vi "sequence.vi"(0 "Elements@IC6":u16[](array[numeric])) -> (1 "Output Array":T2(array[cluster]), 2 "# of layers":i32, 3 "Start/Cancel":bool)   [LabVIEW 2012]
uses:
  elements.gbl
  <vilib>/Utility/VariantDataType/VariantType.lvlib
panel:
  out "Double click":i32
  in  "Clear all":bool
  out "Temp":T1 {"Temp Layer"."T (Å) / D (s)" min=0 format="%.1g"; "Temp Layer"."Elements" items=["none"]}
  in  "Clear layer":bool
  out "error out":errorcluster
  in  "error in (no error)":errorcluster
  in  "Scrollbar":i32(c297)
  in  "Layer Cluster":T3 {"T (Å) / D (s)" min=0 format="%.1g"; "Elements" items=["none"=0, "Se"=2, "Ti"=3, "Sn"=4]}
  in  "Cancel":bool
  in  "Start":bool
  in  "# of repeating units":i32=1 min=1
  in  "Repeats":i32=1 min=1 step=1
  in  "delete_cancel":bool
  in  "add_modify":bool
  in  "down":bool
  in  "up":bool
  in  "Sequence":i32(listbox)=-1
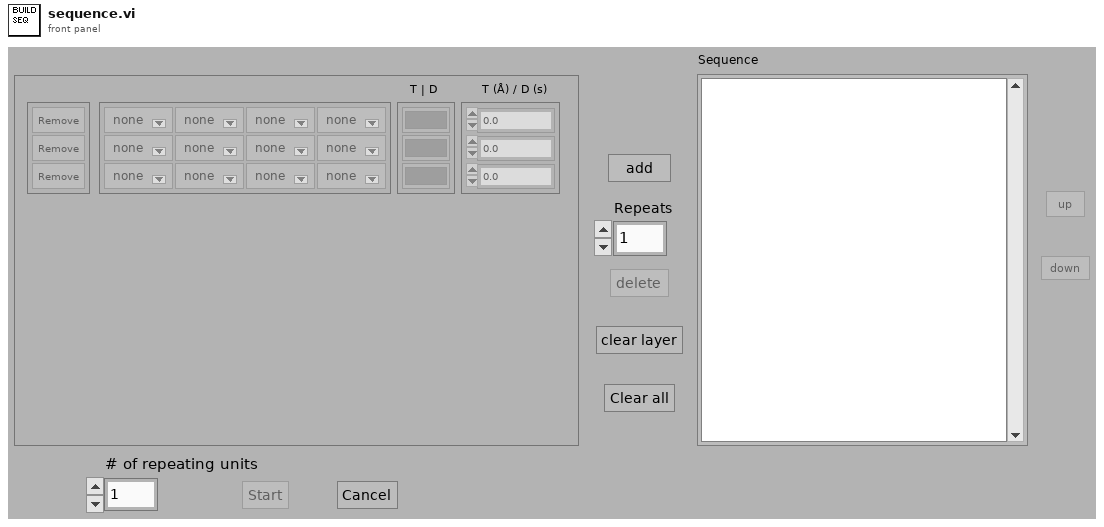
[diagram p1: front panel]
types:
  T1 = cluster{"Temp Layer":cluster{"Remove buttons":bool[], "Elements":u16[][], "T | D":bool[], "T (Å) / D (s)":sgl[]}, "Temp repeats":i32}
  T2 = cluster{"Elements":u16[][], "TD":bool[], "Value":sgl[], "Repeats":i32}[]
  T3 = cluster{"Remove buttons":bool[], "Elements":u16[][], "T | D":bool[], "T (Å) / D (s)":sgl[]}
  T4 = typedef "VariantType.lvlib/Type.ctl" = enum8{"Invalid Type", "Void", "I8", "I16", "I32", "I64", "U8", "U16", "U32", "U64", "Single Float", "Double Float", "Extended Float", "Single Complex", "Double Complex", "Extended Complex", "Enum U8", "Enum U16", "Enum U32", "Enum U64", "Single Float With Unit", "Double Float With Unit", "Extended Float With Unit", "Single Complex with Unit", "Double Complex with Unit", "Extended Complex with Unit", "Boolean", "String", "Path", "Picture", "Tag", "Array", "Cluster", "Variant", "LV Variant", "Waveform", "Timestamp", "Digital Waveform", "Digital Data", "ExpressData", "Refnum", "External Data", "VI", "Poly VI", "LabVIEW Class Instance", "Fixed Point"}
  T5 = cluster{"Layer Cluster":cluster{"Remove buttons":bool[], "Elements":u16[][], "T | D":bool[], "T (Å) / D (s)":sgl[]}, "Repeats":i32}
  T6 = cluster{"Elements":u16[][], "TD":bool[], "Value":sgl[], "Repeats":i32}
  T7 = cluster{bool[], "Elements":u16[][], "TD":bool[], "Value":sgl[]}
  T8 = typedef "LVStringsAndValuesArrayTypeDef_U16.ctl" = cluster{"String":string, "Value":u16}[]
  T9 = cluster{"Elements":u16[][], "T | D":bool[], "T (Å) / D (s)":sgl[]}
  T10 = cluster{"Elements":u16[][], "T|D":bool[], "T (Å) / D (s)":sgl[], "Repeats":i32}
  T11 = cluster{"Elements":u16[][], "T|D":bool[], "T (Å) / D (s)":sgl[], "Repeats":i32}[]
  T12 = cluster{cluster{bool[], u16[][], bool[], sgl[]}, i32}
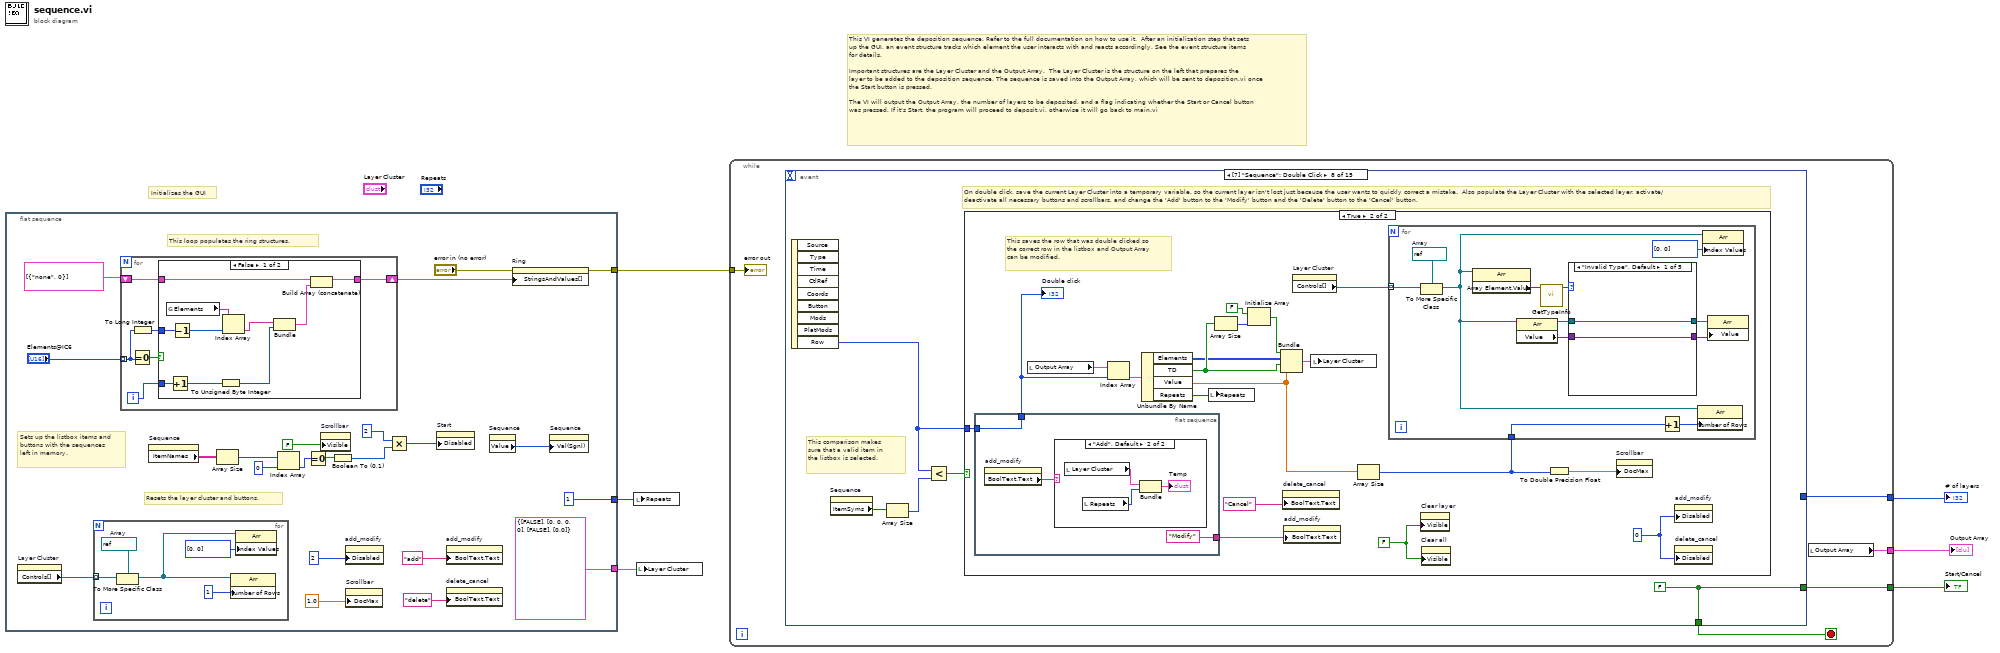
[diagram p0: block diagram]
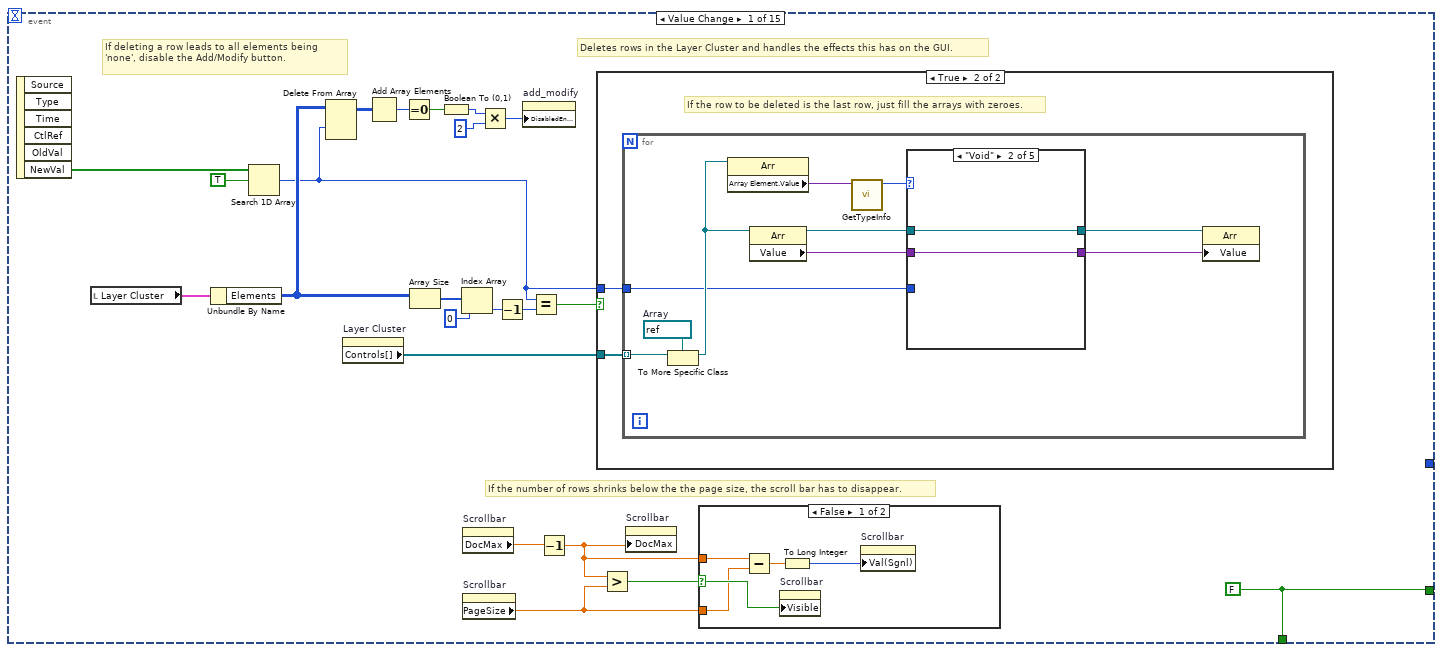
[diagram p2: hidden frame]
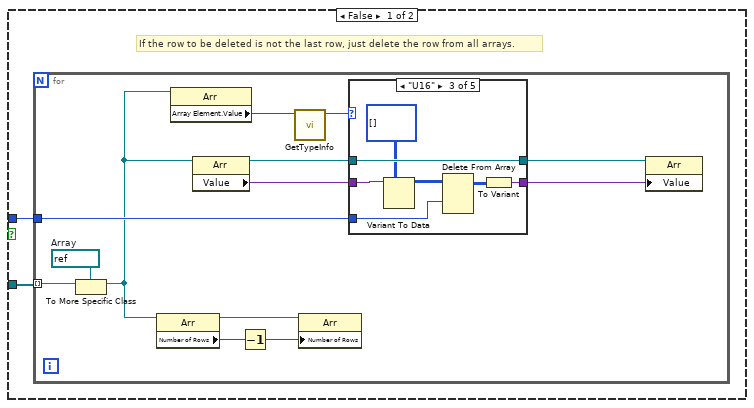
[diagram p4: hidden frame]
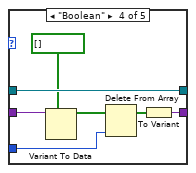
[diagram p7: hidden frame]
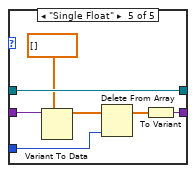
[diagram p8: hidden frame]
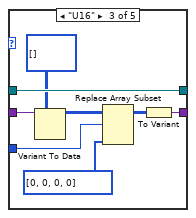
[diagram p10: hidden frame]
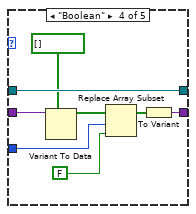
[diagram p11: hidden frame]
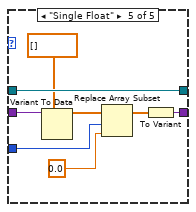
[diagram p12: hidden frame]
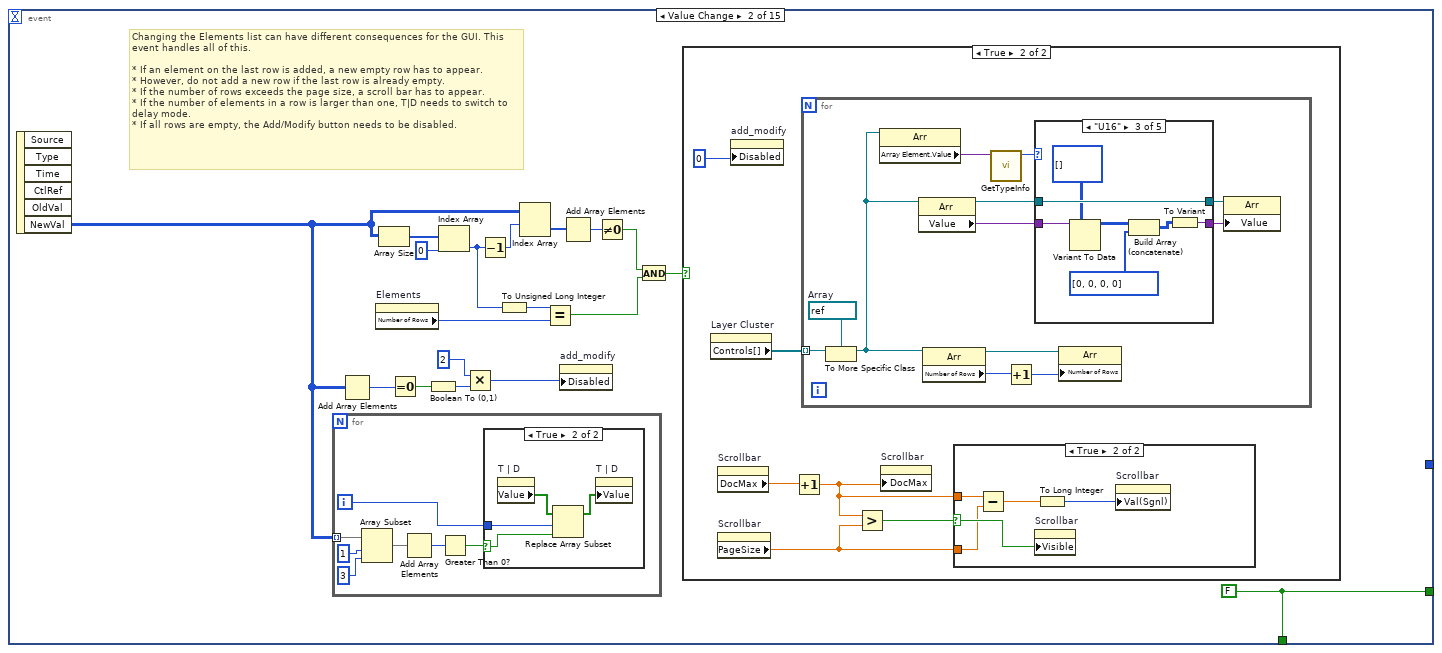
[diagram p13: hidden frame]
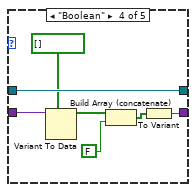
[diagram p19: hidden frame]
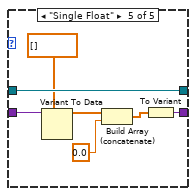
[diagram p20: hidden frame]
diagram:
  # "Initializes the GUI"
  # "This VI generates the deposition sequence. Refer to the full documentation on how to use it.  After an initialization step that sets up the GUI, an event structure tracks which element the user interacts with and reacts accordingly. See the event structure items for details.\n\nImportant structures are the Layer Cluster and the Output Array.  The Layer Cluster is the structure on the left that prepares the layer to be added to the deposition sequence. The sequence is saved into the Output Array, which will be sent to deposition.vi once the Start button is pressed.\n\nThe VI will output the Output Array, the number of layers to be deposited, and a flag indicating whether the Start or Cancel button was pressed. If it's Start, the program will proceed to deposit.vi, otherwise it will go back to main.vi"
  n1 = flat-sequence {
    tunnel: [w28] -> w6
    tunnel: [cluster{bool[], u16[][], bool[], sgl[]} {[FALSE], [[0, 0, 0, 0]], [FALSE], [0.0]}] -> w3
    tunnel: [1] -> w2
    frame #0 {
      # "Sets up the listbox items and buttons with the sequences left in memory."
      # "Resets the layer cluster and buttons."
      # "This loop populates the ring structures."
      n2 = property on="Layer Cluster" class="Clust (strict)"() -> ("Controls[]"=w24:refnum<vi>[])  [unwired: 2 in, 2 out]
      n3 = for {
        tunnel: w24 -> [w32] mode=indexing
        w33 = refnum<vi> refnum  # Array
        n4 = To More Specific Class(target class=w33, reference=w32) -> (specific class reference=w30:refnum<vi>)  [unwired: 1 in, 1 out]
        n5 = property class="Arr"(reference=w30, "Number of Rows"=u32 1) -> ()  [unwired: 1 in, 2 out]
        n6 = property class="Arr"(reference=w30, "Index Values"=u32[] [0, 0]) -> ()  [unwired: 1 in, 2 out]
      }
      n7 = for {
        shift-right: [w38] -> w25
        shift-left: cluster{string, i32}[] [{"none", 0}] -> [w39]
        tunnel: "Elements@IC6" -> [w35] mode=indexing
        i -> [w36]
        n8 = Equal To 0?(x=w35) -> (x = 0?=w37:bool)
        n9 = To Long Integer(number=w35) -> (32bit integer=w34:i32)
        n10 = case shown="False" w37 {
          tunnel: w39 -> [w49 w50]
          tunnel: [w48 w50] -> w38
          tunnel: w36 -> [w47 _]
          tunnel: w34 -> [w45 _]
          frame False {
            n11 = global read "elements.gbl" "Elements"() -> (w46:string[])
            n12 = Increment(x=w47) -> (x+1=w43:i32)
            n13 = Decrement(x=w45) -> (x-1=w40:i32)
            n14 = To Unsigned Byte Integer(number=w43) -> (unsigned 8bit integer=w42:u8)
            n15 = Index Array(array=w46, index=w40) -> (element=w44:string)
            n16 = Bundle("String"=w44, w42) -> (w41:cluster{"String":string, u8})  [unwired: 1 in]
            n17 = Build Array (concatenate)(w49, w41) -> (w48:cluster{"String":string, i32}[])
          }
          frame True {
          }
        }
      }
      n18 = property on="Sequence" class="MCListbox (strict)"() -> ("ItemNames"=w22:string[][])  [unwired: 2 in, 2 out]
      n19 = Array Size(array=w22) -> (size(s)=w21:i32[])
      n20 = Index Array(array=w21, index=0) -> (element=w19:i32)
      n21 = Equal To 0?(x=w19) -> (x = 0?=w18:bool)
      n22 = property on="Scrollbar" class="Scroll (strict)"("Visible"=FALSE) -> ()  [unwired: 2 in, 2 out]
      n23 = Boolean To (0,1)(Boolean=w18) -> (0, 1=w7:i16)
      n24 = property on="add_modify" class="Bool"("Disabled"=2) -> ()  [unwired: 2 in, 2 out]
      n25 = property on="Scrollbar" class="Scroll (strict)"("DocMax"=1.0) -> ()  [unwired: 2 in, 2 out]
      n26 = Multiply(x=i16 2, y=w7) -> (x*y=w16:i16)
      n27 = property on="Start" class="Bool"("Disabled"=w16) -> ()  [unwired: 2 in, 2 out]
      n28 = property on="add_modify" class="Bool"("BoolText.Text"="add") -> ()  [unwired: 2 in, 2 out]
      n29 = property on="delete_cancel" class="Bool"("BoolText.Text"="delete") -> ()  [unwired: 2 in, 2 out]
      n30 = property on="Sequence" class="MCListbox (strict)"() -> ("Value"=w11:i32)  [unwired: 2 in, 2 out]
      n31 = property on="Ring" class="Ring (strict)"(error in="error in (no error)", "StringsAndValues[]"=w25) -> (error out=w28:errorcluster)  [unwired: 1 in, 1 out]
      n32 = property on="Sequence" class="MCListbox (strict)"("Val(Sgnl)"=w11) -> ()  [unwired: 2 in, 2 out]
    }
  }
  n33 = local write "Repeats"(w2) -> ()
  n34 = local write "Layer Cluster"(w3) -> ()
  n35 = while {
    tunnel: w6 -> [w55]
    tunnel: [w54] -> w5
    tunnel: [w51] -> w4
    tunnel: [w52] -> w1
    stop <- w53 stop-if-true
    n36 = event shown="[7] \"Sequence\": Double Click" {
      selector: _ -> [_ _ _ _ _ _ _ _ _ _ _ _ _ _ _]
      dyn-events: _ -> [_ _ _ _ _ _ _ _ _ _ _ _ _ _ _]
      timeout: _ -> [_ _ _ _ _ _ _ _ _ _ _ _ _ _ _]
      tunnel: [w65 w170 w248 w259 w268 "Cancel" w274 w295 w368 w379 w399 w466 w495 w512 w518] -> w53
      tunnel: [w65 w170 w248 w259 w268 w271 w274 w295 w368 w379 w399 w466 w495 w512 w518] -> w54
      tunnel: [_ _ _ _ "# of repeating units" _ _ _ _ _ _ _ _ _ _] -> w51
      event "Layer Cluster.Remove buttons": Value Change {
        w65 = FALSE
        # "If deleting a row leads to all elements being 'none', disable the Add/Modify button."
        # "If the number of rows shrinks below the the page size, the scroll bar has to disappear."
        # "Deletes rows in the Layer Cluster and handles the effects this has on the GUI."
        n37 = event-data() -> ("NewVal"=w76:bool[])  [unwired: 1 in, 5 out]
        n38 = local read "Layer Cluster"() -> (w64:T3)
        n39 = Unbundle By Name(w64) -> ("Elements"=w57:u16[][])
        n40 = Search 1D Array(1D array=w76, element=TRUE) -> (index of element=w56:i32)  [unwired: 1 in]
        n41 = Delete From Array(array=w57, index (row)=w56) -> (array with subset deleted=w58:u16[][])  [unwired: 2 in, 1 out]
        n42 = property on="Layer Cluster" class="Clust (strict)"() -> ("Controls[]"=w75:refnum<vi>[])  [unwired: 2 in, 2 out]
        n43 = Add Array Elements(numeric array=w58) -> (sum=w63:u16)
        n44 = Equal To 0?(x=w63) -> (x = 0?=w62:bool)
        n45 = Array Size(array=w57) -> (size(s)=w74:i32[])
        n46 = Boolean To (0,1)(Boolean=w62) -> (0, 1=w60:i16)
        n47 = Index Array(array=w74, index=0) -> (element=w72:i32)
        n48 = property on="Scrollbar" class="Scroll (strict)"() -> ("DocMax"=w69:dbl)  [unwired: 2 in, 2 out]
        n49 = property on="Scrollbar" class="Scroll (strict)"() -> ("PageSize"=w66:dbl)  [unwired: 2 in, 2 out]
        n50 = Multiply(x=w60, y=2) -> (x*y=w59:i32)
        n51 = Decrement(x=w72) -> (x-1=w70:i32)
        n52 = property on="add_modify" class="Bool"("DisabledEnum"=w59) -> ()  [unwired: 2 in, 2 out]
        n53 = Equal?(x=w56, y=w70) -> (x = y?=w71:bool)
        n54 = Decrement(x=w69) -> (x-1=w68:dbl)
        n55 = case shown="True" w71 {
          tunnel: w75 -> [w84 w124]
          tunnel: w56 -> [w83 w123]
          frame False {
            # "If the row to be deleted is not the last row, just delete the row from all arrays."
            n56 = for {
              tunnel: w84 -> [w93] mode=indexing
              tunnel: w83 -> [w91]
              w97 = refnum<vi> refnum  # Array
              n57 = To More Specific Class(target class=w97, reference=w93) -> (specific class reference=w89:refnum<vi>)  [unwired: 1 in, 1 out]
              n58 = property class="Arr"(reference=w89) -> (reference out=w94:refnum<vi>, "Number of Rows"=w96:u32)  [unwired: 1 in, 1 out]
              n59 = property class="Arr"(reference=w89) -> ("Array Element.Value"=w90:variant)  [unwired: 1 in, 2 out]
              n60 = property class="Arr"(reference=w89) -> (reference out=w86:refnum<vi>, "Value"=w88:variant)  [unwired: 1 in, 1 out]
              n61 = Decrement(x=w96) -> (x-1=w95:u32)
              n62 = call <vilib>:"GetTypeInfo.vi"("Variant"=w90) -> ("Type Enum"=w92:T4)  [unwired: 6 in, 4 out]
              n63 = property class="Arr"(reference=w94, "Number of Rows"=w95) -> ()  [unwired: 1 in, 2 out]
              n64 = case shown="\"U16\"" w92 {
                tunnel: w91 -> [_ _ w102 w114 w121]
                tunnel: w88 -> [w99 w101 w106 w112 w119]
                tunnel: [w99 w101 w107 w109 w118] -> w87
                tunnel: w86 -> [w98 w100 w108 w115 w122]
                tunnel: [w98 w100 w108 w115 w122] -> w85
                frame "Invalid Type", Default {
                }
                frame "Void" {
                }
                frame "U16" {
                  n65 = Variant To Data(type=u16[][] [], Variant=w106) -> (data=w104:u16[][])  [unwired: 1 in, 1 out]
                  n66 = Delete From Array(array=w104, index (row)=w102) -> (array with subset deleted=w105:u16[][])  [unwired: 2 in, 1 out]
                  n67 = To Variant(anything=w105) -> (Variant=w107:variant)
                }
                frame "Boolean" {
                  n68 = Variant To Data(type=bool[] [], Variant=w112) -> (data=w113:bool[])  [unwired: 1 in, 1 out]
                  n69 = Delete From Array(array=w113, index=w114) -> (array with subset deleted=w110:bool[])  [unwired: 1 in, 1 out]
                  n70 = To Variant(anything=w110) -> (Variant=w109:variant)
                }
                frame "Single Float" {
                  n71 = Variant To Data(type=sgl[] [], Variant=w119) -> (data=w120:sgl[])  [unwired: 1 in, 1 out]
                  n72 = Delete From Array(array=w120, index=w121) -> (array with subset deleted=w117:sgl[])  [unwired: 1 in, 1 out]
                  n73 = To Variant(anything=w117) -> (Variant=w118:variant)
                }
              }
              n74 = property class="Arr"(reference=w85, "Value"=w87) -> ()  [unwired: 1 in, 2 out]
            }
          }
          frame True {
            # "If the row to be deleted is the last row, just fill the arrays with zeroes."
            n75 = for {
              tunnel: w124 -> [w127] mode=indexing
              tunnel: w123 -> [w125]
              w128 = refnum<vi> refnum  # Array
              n76 = To More Specific Class(target class=w128, reference=w127) -> (specific class reference=w126:refnum<vi>)  [unwired: 1 in, 1 out]
              n77 = property class="Arr"(reference=w126) -> ("Array Element.Value"=w133:variant)  [unwired: 1 in, 2 out]
              n78 = property class="Arr"(reference=w126) -> (reference out=w129:refnum<vi>, "Value"=w132:variant)  [unwired: 1 in, 1 out]
              n79 = call <vilib>:"GetTypeInfo.vi"("Variant"=w133) -> ("Type Enum"=w134:T4)  [unwired: 6 in, 4 out]
              n80 = case shown="\"Void\"" w134 {
                tunnel: w125 -> [_ _ w140 w153 w161]
                tunnel: w132 -> [w136 w138 w144 w151 w159]
                tunnel: [w136 w138 w145 w148 w158] -> w131
                tunnel: w129 -> [w135 w137 w146 w154 w162]
                tunnel: [w135 w137 w146 w154 w162] -> w130
                frame "Invalid Type", Default {
                }
                frame "Void" {
                }
                frame "U16" {
                  n81 = Variant To Data(type=u16[][] [], Variant=w144) -> (data=w142:u16[][])  [unwired: 1 in, 1 out]
                  n82 = Replace Array Subset(array=w142, new element=u16[] [0, 0, 0, 0], index (row)=w140) -> (w143:u16[][])  [unwired: 1 in]
                  n83 = To Variant(anything=w143) -> (Variant=w145:variant)
                }
                frame "Boolean" {
                  n84 = Variant To Data(type=bool[] [], Variant=w151) -> (data=w152:bool[])  [unwired: 1 in, 1 out]
                  n85 = Replace Array Subset(array=w152, new element=FALSE, index=w153) -> (w149:bool[])
                  n86 = To Variant(anything=w149) -> (Variant=w148:variant)
                }
                frame "Single Float" {
                  n87 = Variant To Data(type=sgl[] [], Variant=w159) -> (data=w160:sgl[])  [unwired: 1 in, 1 out]
                  n88 = Replace Array Subset(array=w160, new element=sgl 0.0, index=w161) -> (w157:sgl[])
                  n89 = To Variant(anything=w157) -> (Variant=w158:variant)
                }
              }
              n90 = property class="Arr"(reference=w130, "Value"=w131) -> ()  [unwired: 1 in, 2 out]
            }
          }
        }
        n91 = Greater?(x=w68, y=w66) -> (0:w67:bool)
        n92 = property on="Scrollbar" class="Scroll (strict)"("DocMax"=w68) -> ()  [unwired: 2 in, 2 out]
        n93 = case shown="False" w67 {
          selector: w67 -> [w82 _]
          tunnel: w68 -> [w80 _]
          tunnel: w66 -> [w79 _]
          frame False {
            n94 = Subtract(x=w80, y=w79) -> (x-y=w78:dbl)
            n95 = property on="Scrollbar" class="Scroll (strict)"("Visible"=w82) -> ()  [unwired: 2 in, 2 out]
            n96 = To Long Integer(number=w78) -> (32bit integer=w81:i32)
            n97 = property on="Scrollbar" class="Scroll (strict)"("Val(Sgnl)"=w81) -> ()  [unwired: 2 in, 2 out]
          }
          frame True {
          }
        }
      }
      event "Layer Cluster.Elements": Value Change {
        w170 = FALSE
        # "Changing the Elements list can have different consequences for the GUI. This event handles all of this.\n\n* If an element on the last row is added, a new empty row has to appear.\n* However, do not add a new row if the last row is already empty.\n* If the number of rows exceeds the page size, a scroll bar has to appear.\n* If the number of elements in a row is larger than one, T|D needs to switch to delay mode.\n* If all rows are empty, the Add/Modify button needs to be disabled."
        n98 = event-data() -> ("NewVal"=w164:u16[][])  [unwired: 1 in, 5 out]
        n99 = for {
          tunnel: w164 -> [w187] mode=indexing
          i -> [w182]
          n100 = Array Subset(array=w187, index=1, length=3) -> (w184:u16[])
          n101 = Add Array Elements(numeric array=w184) -> (sum=w183:u16)
          n102 = Greater Than 0?(x=w183) -> (x > 0?=w181:bool)
          n103 = case shown="True" w181 {
            selector: w181 -> [_ w188]
            tunnel: w182 -> [_ w189]
            frame False {
            }
            frame True {
              n104 = property on="T | D" class="Arr (strict)"() -> ("Value"=w191:bool[])  [unwired: 2 in, 2 out]
              n105 = Replace Array Subset(array=w191, new element=w188, index=w189) -> (w190:bool[])
              n106 = property on="T | D" class="Arr (strict)"("Value"=w190) -> ()  [unwired: 2 in, 2 out]
            }
          }
        }
        n107 = Add Array Elements(numeric array=w164) -> (sum=w169:u16)
        n108 = property on="Elements" class="Arr (strict)"() -> ("Number of Rows"=w171:u32)  [unwired: 2 in, 2 out]
        n109 = Array Size(array=w164) -> (size(s)=w180:i32[])
        n110 = Equal To 0?(x=w169) -> (x = 0?=w168:bool)
        n111 = Boolean To (0,1)(Boolean=w168) -> (0, 1=w167:i16)
        n112 = Index Array(array=w180, index=0) -> (element=w172:i32)
        n113 = Multiply(x=i16 2, y=w167) -> (x*y=w165:i16)
        n114 = Decrement(x=w172) -> (x-1=w176:i32)
        n115 = To Unsigned Long Integer(number=w172) -> (unsigned 32bit integer=w163:u32)
        n116 = Index Array(array=w164, index (row)=w176) -> (element=w178:u16[])  [unwired: 1 in]
        n117 = Equal?(x=w163, y=w171) -> (x = y?=w173:bool)
        n118 = property on="add_modify" class="Bool"("Disabled"=w165) -> ()  [unwired: 2 in, 2 out]
        n119 = Add Array Elements(numeric array=w178) -> (sum=w177:u16)
        n120 = Not Equal To 0?(x=w177) -> (x != 0?=w174:bool)
        n121 = And(x=w174, y=w173) -> (x .and. y?=w175:bool)
        n122 = case shown="True" w175 {
          frame False {
            # "Last row is empty, so do not add another empty row."
          }
          frame True {
            n123 = property on="Layer Cluster" class="Clust (strict)"() -> ("Controls[]"=w197:refnum<vi>[])  [unwired: 2 in, 2 out]
            n124 = property on="Scrollbar" class="Scroll (strict)"() -> ("DocMax"=w196:dbl)  [unwired: 2 in, 2 out]
            n125 = property on="Scrollbar" class="Scroll (strict)"() -> ("PageSize"=w193:dbl)  [unwired: 2 in, 2 out]
            n126 = property on="add_modify" class="Bool"("Disabled"=u16 0) -> ()  [unwired: 2 in, 2 out]
            n127 = Increment(x=w196) -> (x+1=w195:dbl)
            n128 = for {
              tunnel: w197 -> [w214] mode=indexing
              w213 = refnum<vi> refnum  # Array
              n129 = To More Specific Class(target class=w213, reference=w214) -> (specific class reference=w204:refnum<vi>)  [unwired: 1 in, 1 out]
              n130 = property class="Arr"(reference=w204) -> ("Array Element.Value"=w203:variant)  [unwired: 1 in, 2 out]
              n131 = property class="Arr"(reference=w204) -> (reference out=w207:refnum<vi>, "Value"=w206:variant)  [unwired: 1 in, 1 out]
              n132 = property class="Arr"(reference=w204) -> (reference out=w212:refnum<vi>, "Number of Rows"=w210:u32)  [unwired: 1 in, 1 out]
              n133 = call <vilib>:"GetTypeInfo.vi"("Variant"=w203) -> ("Type Enum"=w205:T4)  [unwired: 6 in, 4 out]
              n134 = Increment(x=w210) -> (x+1=w211:u32)
              n135 = case shown="\"U16\"" w205 {
                tunnel: w206 -> [w216 w218 w223 w230 w237]
                tunnel: [w216 w218 w224 w227 w236] -> w208
                tunnel: w207 -> [w215 w217 w225 w232 w239]
                tunnel: [w215 w217 w225 w232 w239] -> w209
                frame "Invalid Type", Default {
                }
                frame "Void" {
                }
                frame "U16" {
                  n136 = Variant To Data(type=u16[][] [], Variant=w223) -> (data=w219:u16[][])  [unwired: 1 in, 1 out]
                  n137 = Build Array (concatenate)(w219, u16[] [0, 0, 0, 0]) -> (w222:u16[][])
                  n138 = To Variant(anything=w222) -> (Variant=w224:variant)
                }
                frame "Boolean" {
                  n139 = Variant To Data(type=bool[] [], Variant=w230) -> (data=w231:bool[])  [unwired: 1 in, 1 out]
                  n140 = Build Array (concatenate)(w231, FALSE) -> (w228:bool[])
                  n141 = To Variant(anything=w228) -> (Variant=w227:variant)
                }
                frame "Single Float" {
                  n142 = Variant To Data(type=sgl[] [], Variant=w237) -> (data=w238:sgl[])  [unwired: 1 in, 1 out]
                  n143 = Build Array (concatenate)(w238, sgl 0.0) -> (w235:sgl[])
                  n144 = To Variant(anything=w235) -> (Variant=w236:variant)
                }
              }
              n145 = property class="Arr"(reference=w212, "Number of Rows"=w211) -> ()  [unwired: 1 in, 2 out]
              n146 = property class="Arr"(reference=w209, "Value"=w208) -> ()  [unwired: 1 in, 2 out]
            }
            n147 = Greater?(x=w195, y=w193) -> (0:w194:bool)
            n148 = property on="Scrollbar" class="Scroll (strict)"("DocMax"=w195) -> ()  [unwired: 2 in, 2 out]
            n149 = case shown="True" w194 {
              selector: w194 -> [_ w202]
              tunnel: w195 -> [_ w201]
              tunnel: w193 -> [_ w198]
              frame False {
              }
              frame True {
                n150 = Subtract(x=w201, y=w198) -> (x-y=w199:dbl)
                n151 = property on="Scrollbar" class="Scroll (strict)"("Visible"=w202) -> ()  [unwired: 2 in, 2 out]
                n152 = To Long Integer(number=w199) -> (32bit integer=w200:i32)
                n153 = property on="Scrollbar" class="Scroll (strict)"("Val(Sgnl)"=w200) -> ()  [unwired: 2 in, 2 out]
              }
            }
          }
        }
      }
      event "Layer Cluster.T | D": Value Change {
        w248 = FALSE
        # "Prevents going to thickness mode when more than one element is in the layer."
        n154 = event-data() -> ("OldVal"=w253:bool[], "NewVal"=w252:bool[])  [unwired: 1 in, 4 out]
        n155 = Not Equal?(x=w253, y=w252) -> (x != y?=w251:bool[])
        n156 = Search 1D Array(1D array=w251, element=TRUE) -> (index of element=w246:i32)  [unwired: 1 in]
        n157 = local read "Layer Cluster"() -> (w249:T3)
        n158 = Unbundle By Name(w249) -> ("Elements"=w247:u16[][])
        n159 = Index Array(array=w247, index (row)=w246) -> (element=w245:u16[])  [unwired: 1 in]
        n160 = Not Equal To 0?(x=w245) -> (x != 0?=w244:bool[])
        n161 = Boolean To (0,1)(Boolean=w244) -> (0, 1=w243:i16[])
        n162 = Add Array Elements(numeric array=w243) -> (sum=w241:i16)
        n163 = Less?(x=i16 1, y=w241) -> (x < y?=w242:bool)
        n164 = case shown="True" w242 {
          selector: w242 -> [_ w254]
          tunnel: w246 -> [_ w255]
          frame False {
          }
          frame True {
            n165 = property on="T | D" class="Arr (strict)"() -> ("Value"=w257:bool[])  [unwired: 2 in, 2 out]
            n166 = Replace Array Subset(array=w257, new element=w254, index=w255) -> (w256:bool[])
            n167 = property on="T | D" class="Arr (strict)"("Value"=w256) -> ()  [unwired: 2 in, 2 out]
          }
        }
      }
      event "Scrollbar": Value Change {
        w259 = FALSE
        # "Moves the layer cluster with the scrollbar."
        n168 = event-data() -> ("NewVal"=w258:i32)  [unwired: 1 in, 5 out]
        n169 = property on="Layer Cluster" class="Clust (strict)"() -> ("Controls[]"=w262:refnum<vi>[])  [unwired: 2 in, 2 out]
        n170 = Build Array(w258, 0) -> (w260:i32[])
        n171 = for {
          tunnel: w262 -> [w266] mode=indexing
          tunnel: w260 -> [w264]
          w267 = refnum<vi> refnum  # Array
          n172 = To Unsigned Long Integer(number=w264) -> (unsigned 32bit integer=w263:u32[])
          n173 = To More Specific Class(target class=w267, reference=w266) -> (specific class reference=w265:refnum<vi>)  [unwired: 1 in, 1 out]
          n174 = property class="Arr"(reference=w265, "Index Values"=w263) -> ()  [unwired: 1 in, 2 out]
        }
      }
      event "Start": Value Change {
        w268 = TRUE
        # "Quits the VI and sends a True (Start) signal and the number of layers to main.vi"
        n175 = event-data() -> ()  [unwired: 1 in, 6 out]
      }
      event "Cancel": Value Change {
        # "Quits the VI and sends a False (Cancel) signal to main.vi"
        n176 = event-data() -> ()  [unwired: 1 in, 6 out]
        n177 = Not(x="Cancel") -> (.not. x?=w271:bool)
      }
      event "Sequence": Value Change {
        w274 = FALSE
        # "Activates/dectivates buttons, depending on which item in the listbox is selected.\n\n0: First item selected, disable the 'up' button.\n< 0: No item selected, disable the 'delete' button.\n= length of items - 1: Last item selected, disable 'down' button."
        n178 = event-data() -> ("NewVal"=w275:i32)  [unwired: 1 in, 5 out]
        n179 = property on="Sequence" class="MCListbox (strict)"() -> ("ItemSyms"=w280:i32[])  [unwired: 2 in, 2 out]
        n180 = Array Size(array=w280) -> (size(s)=w272:i32)
        n181 = Decrement(x=w272) -> (x-1=w273:i32)
        n182 = Equal To 0?(x=w275) -> (x = 0?=w283:bool)
        n183 = Less Than 0?(x=w275) -> (x < 0?=w277:bool)
        n184 = Equal?(x=w275, y=w273) -> (x = y?=w281:bool)
        n185 = Or(x=w283, y=w277) -> (x .or. y?=w284:bool)
        n186 = Or(x=w277, y=w281) -> (x .or. y?=w282:bool)
        n187 = Boolean To (0,1)(Boolean=w277) -> (0, 1=w278:i16)
        n188 = Boolean To (0,1)(Boolean=w284) -> (0, 1=w290:i16)
        n189 = Boolean To (0,1)(Boolean=w282) -> (0, 1=w287:i16)
        n190 = Multiply(x=i16 2, y=w290) -> (x*y=w288:i16)
        n191 = Multiply(x=i16 2, y=w278) -> (x*y=w276:i16)
        n192 = Multiply(x=i16 2, y=w287) -> (x*y=w285:i16)
        n193 = property on="up" class="Bool"("Disabled"=w288) -> ()  [unwired: 2 in, 2 out]
        n194 = property on="delete_cancel" class="Bool"("Disabled"=w276) -> ()  [unwired: 2 in, 2 out]
        n195 = property on="down" class="Bool"("Disabled"=w285) -> ()  [unwired: 2 in, 2 out]
      }
      event "Sequence": Double Click {
        w295 = FALSE
        # "On double click, save the current Layer Cluster into a temporary variable, so the current layer isn't lost just because the user wants to quickly correct a mistake.  Also populate the Layer Cluster with the selected layer, activate/deactivate all necessary buttons and scrollbars, and change the 'Add' button to the 'Modify' button and the 'Delete' button to the 'Cancel' button."
        # "This comparison makes sure that a valid item in the listbox is selected."
        n196 = event-data() -> ("Row"=w291:i32)  [unwired: 1 in, 8 out]
        n197 = property on="Sequence" class="MCListbox (strict)"() -> ("ItemSyms"=w294:i32[])  [unwired: 2 in, 2 out]
        n198 = Array Size(array=w294) -> (size(s)=w292:i32)
        n199 = Less?(x=w291, y=w292) -> (x < y?=w293:bool)
        n200 = case shown="True" w293 {
          tunnel: w291 -> [_ w302]
          frame False {
          }
          frame True {
            w305 = FALSE
            w298 = 0
            # "This saves the row that was double clicked so the correct row in the listbox and Output Array can be modified."
            n201 = flat-sequence {
              tunnel: w302 -> [w353]
              tunnel: [w353] -> w297
              tunnel: ["Modify"] -> w296
              frame #0 {
                n202 = property on="add_modify" class="Bool"() -> ("BoolText.Text"=w354:string)  [unwired: 2 in, 2 out]
                n203 = case shown="\"Add\", Default" w354 {
                  frame "Modify" {
                  }
                  frame "Add", Default {
                    n204 = local read "Layer Cluster"() -> (w356:T3)
                    n205 = local read "Repeats"() -> (w355:i32)
                    n206 = Bundle("Layer Cluster"=w356, "Repeats"=w355) -> (→"Temp":T5)  [unwired: 1 in]
                  }
                }
              }
            }
            n207 = local read "Output Array"() -> (w313:T2)
            n208 = Index Array(array=w313, index=w297) -> (element=w312:T6)
            n209 = Unbundle By Name(w312) -> ("Elements"=w301:u16[][], "TD"=w306:bool[], "Value"=w304:sgl[], "Repeats"=w311:i32)
            n210 = local write "Repeats"(w311) -> ()
            n211 = Array Size(array=w306) -> (size(s)=w309:i32)
            n212 = Initialize Array(FALSE, w309) -> (w308:bool[])
            n213 = Bundle(w308, "Elements"=w301, "TD"=w306, "Value"=w304) -> (w307:T7)  [unwired: 1 in]
            n214 = property on="delete_cancel" class="Bool"("BoolText.Text"="Cancel") -> ()  [unwired: 2 in, 2 out]
            n215 = property on="add_modify" class="Bool"("BoolText.Text"=w296) -> ()  [unwired: 2 in, 2 out]
            n216 = property on="Layer Cluster" class="Clust (strict)"() -> ("Controls[]"=w300:refnum<vi>[])  [unwired: 2 in, 2 out]
            n217 = local write "Layer Cluster"(w307) -> ()
            n218 = Array Size(array=w304) -> (size(s)=w299:i32)
            n219 = for {
              tunnel: w300 -> [w325] mode=indexing
              tunnel: w299 -> [w323]
              w326 = refnum<vi> refnum  # Array
              n220 = To More Specific Class(target class=w326, reference=w325) -> (specific class reference=w315:refnum<vi>)  [unwired: 1 in, 1 out]
              n221 = property class="Arr"(reference=w315) -> ("Array Element.Value"=w317:variant)  [unwired: 1 in, 2 out]
              n222 = property class="Arr"(reference=w315) -> (reference out=w318:refnum<vi>, "Value"=w319:variant)  [unwired: 1 in, 1 out]
              n223 = call <vilib>:"GetTypeInfo.vi"("Variant"=w317) -> ("Type Enum"=w316:T4)  [unwired: 6 in, 4 out]
              n224 = case shown="\"Invalid Type\", Default" w316 {
                tunnel: w319 -> [w328 w330 w335 w342 w349]
                tunnel: [w328 w330 w336 w339 w348] -> w320
                tunnel: w318 -> [w327 w329 w337 w344 w351]
                tunnel: [w327 w329 w337 w344 w351] -> w321
                frame "Invalid Type", Default {
                }
                frame "Void" {
                }
                frame "U16" {
                  n225 = Variant To Data(type=u16[][] [], Variant=w335) -> (data=w333:u16[][])  [unwired: 1 in, 1 out]
                  n226 = Build Array (concatenate)(w333, u16[] [0, 0, 0, 0]) -> (w334:u16[][])
                  n227 = To Variant(anything=w334) -> (Variant=w336:variant)
                }
                frame "Boolean" {
                  n228 = Variant To Data(type=bool[] [], Variant=w342) -> (data=w343:bool[])  [unwired: 1 in, 1 out]
                  n229 = Build Array (concatenate)(w343, FALSE) -> (w340:bool[])
                  n230 = To Variant(anything=w340) -> (Variant=w339:variant)
                }
                frame "Single Float" {
                  n231 = Variant To Data(type=sgl[] [], Variant=w349) -> (data=w350:sgl[])  [unwired: 1 in, 1 out]
                  n232 = Build Array (concatenate)(w350, sgl 0.0) -> (w347:sgl[])
                  n233 = To Variant(anything=w347) -> (Variant=w348:variant)
                }
              }
              n234 = Increment(x=w323) -> (x+1=w322:i32)
              n235 = property class="Arr"(reference=w315, "Number of Rows"=w322) -> ()  [unwired: 1 in, 2 out]
              n236 = property class="Arr"(reference=w315, "Index Values"=i32[] [0, 0]) -> ()  [unwired: 1 in, 2 out]
              n237 = property class="Arr"(reference=w321, "Value"=w320) -> ()  [unwired: 1 in, 2 out]
            }
            n238 = property on="Clear layer" class="Bool"("Visible"=w305) -> ()  [unwired: 2 in, 2 out]
            n239 = property on="Clear all" class="Bool"("Visible"=w305) -> ()  [unwired: 2 in, 2 out]
            n240 = To Double Precision Float(number=w299) -> (double precision float=w303:dbl)
            n241 = property on="Scrollbar" class="Scroll (strict)"("DocMax"=w303) -> ()  [unwired: 2 in, 2 out]
            n242 = property on="add_modify" class="Bool"("Disabled"=w298) -> ()  [unwired: 2 in, 2 out]
            n243 = property on="delete_cancel" class="Bool"("Disabled"=w298) -> ()  [unwired: 2 in, 2 out]
            "Double click" <- w297
          }
        }
      }
      event "up": Value Change {
        w368 = FALSE
        # "Moves the selected layer up in the listbox and in the Output Array, and triggers the \"Sequence: Value Change\" event to activate/deactivate the 'up' button if necessary."
        n244 = event-data() -> ()  [unwired: 1 in, 6 out]
        n245 = local read "Output Array"() -> (w367:T2)
        n246 = property on="Sequence" class="MCListbox (strict)"() -> ("ItemNames"=w361:string[][])  [unwired: 2 in, 2 out]
        n247 = property on="Sequence" class="MCListbox (strict)"() -> ("Value"=w359:i32)  [unwired: 2 in, 2 out]
        n248 = Delete From Array(array=w361, index (row)=w359) -> (deleted portion=w363:string[], array with subset deleted=w362:string[][])  [unwired: 2 in]
        n249 = Delete From Array(array=w367, index=w359) -> (deleted portion=w366:T6, array with subset deleted=w365:T2)  [unwired: 1 in]
        n250 = Decrement(x=w359) -> (x-1=w358:i32)
        n251 = Insert Into Array(array=w362, index (row)=w358, new element=w363) -> (w360:string[][])  [unwired: 1 in]
        n252 = Insert Into Array(array=w365, index=w358, new element=w366) -> (w364:T2)
        n253 = property on="Sequence" class="MCListbox (strict)"("Val(Sgnl)"=w358) -> ()  [unwired: 2 in, 2 out]
        n254 = local write "Output Array"(w364) -> ()
        n255 = property on="Sequence" class="MCListbox (strict)"("ItemNames"=w360) -> ()  [unwired: 2 in, 2 out]
      }
      event "down": Value Change {
        w379 = FALSE
        # "Moves the selected layer down in the listbox and in the Output Array, and triggers the \"Sequence: Value Change\" event to activate/deactivate the 'down' button if necessary."
        n256 = event-data() -> ()  [unwired: 1 in, 6 out]
        n257 = local read "Output Array"() -> (w372:T2)
        n258 = property on="Sequence" class="MCListbox (strict)"() -> ("ItemNames"=w377:string[][])  [unwired: 2 in, 2 out]
        n259 = property on="Sequence" class="MCListbox (strict)"() -> ("Value"=w369:i32)  [unwired: 2 in, 2 out]
        n260 = Increment(x=w369) -> (x+1=w370:i32)
        n261 = Delete From Array(array=w377, index (row)=w369) -> (deleted portion=w375:string[], array with subset deleted=w376:string[][])  [unwired: 2 in]
        n262 = Delete From Array(array=w372, index=w369) -> (deleted portion=w373:T6, array with subset deleted=w374:T2)  [unwired: 1 in]
        n263 = Insert Into Array(array=w376, index (row)=w370, new element=w375) -> (w378:string[][])  [unwired: 1 in]
        n264 = Insert Into Array(array=w374, index=w370, new element=w373) -> (w371:T2)
        n265 = property on="Sequence" class="MCListbox (strict)"("Val(Sgnl)"=w370) -> ()  [unwired: 2 in, 2 out]
        n266 = local write "Output Array"(w371) -> ()
        n267 = property on="Sequence" class="MCListbox (strict)"("ItemNames"=w378) -> ()  [unwired: 2 in, 2 out]
      }
      event "add_modify": Value Change {
        w399 = FALSE
        # "Sends the layer cluster to the format_layer.vi to process. The result will either modify or append to the Output Array, depending on whether the 'Modify' or 'Add' button is active."
        n268 = event-data() -> ()  [unwired: 1 in, 6 out]
        n269 = local read "Layer Cluster"() -> (w385:T3)
        n270 = property on="Ring" class="Ring (strict)"() -> ("StringsAndValues[]"=w380:T8)  [unwired: 2 in, 2 out]
        n271 = Unbundle By Name(w385) -> ("Elements"=w384:u16[][], "T | D"=w383:bool[], "T (Å) / D (s)"=w382:sgl[])
        n272 = local read "Repeats"() -> (w392:i32)
        n273 = Bundle("Elements"=w384, "T | D"=w383, "T (Å) / D (s)"=w382) -> (w381:T9)  [unwired: 1 in]
        n274 = call "format_layer.vi"("Repeats"=w392, "Input cluster"=w381, "Source"=w380) -> ("Output cluster"=w397:T10, "Listbox text"=w398:string[])
        n275 = Unbundle By Name(w397) -> ("Elements"=w389:u16[][], "T (Å) / D (s)"=w396:sgl[])
        n276 = local read "Double click"() -> (w386:i32)
        n277 = Add Array Elements(numeric array=w389) -> (sum=w390:u16)
        n278 = Search 1D Array(1D array=w396, element=sgl 0.0) -> (index of element=w393:i32)  [unwired: 1 in]
        n279 = Equal?(x=-1, y=w393) -> (x = y?=w387:bool)
        n280 = Not Equal To 0?(x=w390) -> (x != 0?=w388:bool)
        n281 = And(x=w388, y=w387) -> (x .and. y?=w391:bool)
        n282 = case shown="True" w391 {
          tunnel: w386 -> [_ w418]
          tunnel: w398 -> [_ w416]
          tunnel: w397 -> [_ w415]
          tunnel: w388 -> [w404 _]
          tunnel: w387 -> [w403 _]
          frame False {
            # "If all elements are 'none', or the thickness/delay value is zero, don't do anything."
            n283 = case shown="False" w404 {
              tunnel: [w413 ""] -> w402
              frame False {
                n284 = Concatenate Strings("No elements selected.", "\r\n") -> (w413:string)
              }
              frame True {
              }
            }
            n285 = case shown="False" w403 {
              tunnel: [w409 ""] -> w401
              frame False {
                n286 = Concatenate Strings("At least one layer has a thickness/delay value of zero.", "\r\n") -> (w409:string)
              }
              frame True {
              }
            }
            n287 = Concatenate Strings("Error: can't add repeat unit to sequence.", "\r\n", w402, w401) -> (w400:string)
            n288 = One Button Dialog(message=w400) -> ()  [unwired: 1 in, 1 out]
          }
          frame True {
            n289 = property on="add_modify" class="Bool"() -> ("BoolText.Text"=w417:string)  [unwired: 2 in, 2 out]
            n290 = case shown="\"Add\", Default" w417 {
              tunnel: w415 -> [w420 w439]
              tunnel: w416 -> [w419 w440]
              tunnel: w418 -> [_ w438]
              frame "Add", Default {
                # "Append the output of the format_layer.vi to the listbox and the Output Array and reset the Layer Cluster."
                n291 = flat-sequence {
                  tunnel: w420 -> [w424]
                  tunnel: w419 -> [w423]
                  frame #0 {
                    n292 = local read "Output Array"() -> (w426:T2)
                    n293 = property on="Sequence" class="MCListbox (strict)"() -> ("ItemNames"=w422:string[][])  [unwired: 2 in, 2 out]
                    n294 = Build Array (concatenate)(w422, w423) -> (w421:string[][])
                    n295 = Build Array (concatenate)(w426, w424) -> (w425:T11)
                    n296 = local write "Output Array"(w425) -> ()
                    n297 = property on="Sequence" class="MCListbox (strict)"("ItemNames"=w421) -> ()  [unwired: 2 in, 2 out]
                  }
                  frame #1 {
                    n298 = property on="Sequence" class="MCListbox (strict)"() -> ("Value"=w428:i32)  [unwired: 2 in, 2 out]
                    n299 = property on="Layer Cluster" class="Clust (strict)"() -> ("Controls[]"=w429:refnum<vi>[])  [unwired: 2 in, 2 out]
                    n300 = for {
                      tunnel: w429 -> [w436] mode=indexing
                      w437 = refnum<vi> refnum  # Array
                      n301 = To More Specific Class(target class=w437, reference=w436) -> (specific class reference=w434:refnum<vi>)  [unwired: 1 in, 1 out]
                      n302 = property class="Arr"(reference=w434, "Number of Rows"=u32 1) -> ()  [unwired: 1 in, 2 out]
                      n303 = property class="Arr"(reference=w434, "Index Values"=u32[] [0, 0]) -> ()  [unwired: 1 in, 2 out]
                    }
                    n304 = property on="Sequence" class="MCListbox (strict)"("Val(Sgnl)"=w428) -> ()  [unwired: 2 in, 2 out]
                    n305 = local write "Layer Cluster"(cluster{bool[], u16[][], bool[], sgl[]} {[FALSE], [[0, 0, 0, 0]], [FALSE], [0.0]}) -> ()
                    n306 = local write "Repeats"(1) -> ()
                    n307 = property on="Start" class="Bool"("Disabled"=0) -> ()  [unwired: 2 in, 2 out]
                    n308 = property on="add_modify" class="Bool"("Disabled"=2) -> ()  [unwired: 2 in, 2 out]
                  }
                }
              }
              frame "Modify" {
                # "Replace the modified layer with the new layer in the listbox and Output array. Then, repopulate the Layer Cluster with the cluster saved in the Temp variable and change the 'Modify' button to the 'Add' button and the 'Cancel' button to the 'Delete' button."
                n309 = flat-sequence {
                  tunnel: w440 -> [w448]
                  tunnel: w439 -> [w447]
                  tunnel: w438 -> [w442]
                  tunnel: w438 -> [w441]
                  frame #0 {
                    n310 = local read "Output Array"() -> (w446:T2)
                    n311 = property on="Sequence" class="MCListbox (strict)"() -> ("ItemNames"=w444:string[][])  [unwired: 2 in, 2 out]
                    n312 = Replace Array Subset(array=w444, new element=w448, index (row)=w442) -> (w443:string[][])  [unwired: 1 in]
                    n313 = Replace Array Subset(array=w446, new element=w447, index=w441) -> (w445:T2)
                    n314 = local write "Output Array"(w445) -> ()
                    n315 = property on="Sequence" class="MCListbox (strict)"("ItemNames"=w443) -> ()  [unwired: 2 in, 2 out]
                  }
                  frame #1 {
                    w451 = TRUE
                    n316 = property on="Layer Cluster" class="Clust (strict)"() -> ("Controls[]"=w455:refnum<vi>[])  [unwired: 2 in, 2 out]
                    n317 = local read "Temp"() -> (w457:T1)
                    n318 = property on="Clear layer" class="Bool"("Visible"=w451) -> ()  [unwired: 2 in, 2 out]
                    n319 = property on="Clear all" class="Bool"("Visible"=w451) -> ()  [unwired: 2 in, 2 out]
                    n320 = Unbundle(w457) -> ("Temp Layer"=w454:T3, "Temp repeats"=w458:i32)
                    n321 = Unbundle By Name(w454) -> ("Remove buttons"=w453:bool[])
                    n322 = local write "Layer Cluster"(w454) -> ()
                    n323 = local write "Repeats"(w458) -> ()
                    n324 = Array Size(array=w453) -> (size(s)=w449:i32)
                    n325 = for {
                      tunnel: w455 -> [w463] mode=indexing
                      tunnel: w449 -> [w460]
                      w464 = refnum<vi> refnum  # Array
                      n326 = To More Specific Class(target class=w464, reference=w463) -> (specific class reference=w462:refnum<vi>)  [unwired: 1 in, 1 out]
                      n327 = To Unsigned Long Integer(number=w460) -> (unsigned 32bit integer=w459:u32)
                      n328 = property class="Arr"(reference=w462, "Index Values"=u32[] [0, 0]) -> ()  [unwired: 1 in, 2 out]
                      n329 = property class="Arr"(reference=w462, "Number of Rows"=w459) -> ()  [unwired: 1 in, 2 out]
                    }
                    n330 = To Double Precision Float(number=w449) -> (double precision float=w450:dbl)
                    n331 = property on="add_modify" class="Bool"("BoolText.Text"="add") -> ()  [unwired: 2 in, 2 out]
                    n332 = property on="delete_cancel" class="Bool"("BoolText.Text"="delete") -> ()  [unwired: 2 in, 2 out]
                    n333 = property on="Scrollbar" class="Scroll (strict)"("DocMax"=w450) -> ()  [unwired: 2 in, 2 out]
                  }
                }
              }
            }
          }
        }
      }
      event "delete_cancel": Value Change {
        w466 = FALSE
        # "Delete the layer or cancels changes to a layer, depending on which button is active."
        n334 = event-data() -> ()  [unwired: 1 in, 6 out]
        n335 = property on="delete_cancel" class="Bool"() -> ("BoolText.Text"=w465:string)  [unwired: 2 in, 2 out]
        n336 = case shown="\"Cancel\"" w465 {
          frame "Delete", Default {
            # "Deletes a layer from the Output Array and the listbox. If this creates an empty Output array, disable the Start button. Trigger the \"Sequence: Value Change\" event afterwards to disable the 'up', 'down', or 'delete' button if necessary."
            n337 = flat-sequence {
              frame #0 {
                n338 = local read "Output Array"() -> (w476:T2)
                n339 = property on="Sequence" class="MCListbox (strict)"() -> ("ItemNames"=w475:string[][])  [unwired: 2 in, 2 out]
                n340 = property on="Sequence" class="MCListbox (strict)"() -> ("Value"=w473:i32)  [unwired: 2 in, 2 out]
                n341 = Delete From Array(array=w476, index=w473) -> (array with subset deleted=w472:T2)  [unwired: 1 in, 1 out]
                n342 = Delete From Array(array=w475, index (row)=w473) -> (array with subset deleted=w474:string[][])  [unwired: 2 in, 1 out]
                n343 = local write "Output Array"(w472) -> ()
                n344 = property on="Sequence" class="MCListbox (strict)"("ItemNames"=w474) -> ()  [unwired: 2 in, 2 out]
                n345 = Array Size(array=w472) -> (size(s)=w471:i32)
                n346 = Equal To 0?(x=w471) -> (x = 0?=w467:bool)
                n347 = Boolean To (0,1)(Boolean=w467) -> (0, 1=w468:i16)
                n348 = Multiply(x=i16 2, y=w468) -> (x*y=w470:i16)
                n349 = property on="Start" class="Bool"("Disabled"=w470) -> ()  [unwired: 2 in, 2 out]
              }
              frame #1 {
                n350 = property on="Sequence" class="MCListbox (strict)"() -> ("Value"=w477:i32)  [unwired: 2 in, 2 out]
                n351 = property on="Sequence" class="MCListbox (strict)"("Val(Sgnl)"=w477) -> ()  [unwired: 2 in, 2 out]
              }
            }
          }
          frame "Cancel" {
            w483 = TRUE
            # "Revert all changes by repopulating the layer cluster with the Temp variable. Change the 'Modify' button back to the 'Add' button and the 'Cancel' button to the 'Delete' button."
            n352 = property on="add_modify" class="Bool"("BoolText.Text"="add") -> ()  [unwired: 2 in, 2 out]
            n353 = property on="delete_cancel" class="Bool"("BoolText.Text"="delete") -> ()  [unwired: 2 in, 2 out]
            n354 = property on="Layer Cluster" class="Clust (strict)"() -> ("Controls[]"=w482:refnum<vi>[])  [unwired: 2 in, 2 out]
            n355 = local read "Temp"() -> (w486:T1)
            n356 = property on="Clear layer" class="Bool"("Visible"=w483) -> ()  [unwired: 2 in, 2 out]
            n357 = property on="Clear all" class="Bool"("Visible"=w483) -> ()  [unwired: 2 in, 2 out]
            n358 = Unbundle(w486) -> ("Temp Layer"=w480:T3, "Temp repeats"=w487:i32)
            n359 = local write "Layer Cluster"(w480) -> ()
            n360 = Unbundle By Name(w480) -> ("Remove buttons"=w481:bool[])
            n361 = local write "Repeats"(w487) -> ()
            n362 = Array Size(array=w481) -> (size(s)=w479:i32)
            n363 = for {
              tunnel: w482 -> [w492] mode=indexing
              tunnel: w479 -> [w489]
              w493 = refnum<vi> refnum  # Array
              n364 = To More Specific Class(target class=w493, reference=w492) -> (specific class reference=w491:refnum<vi>)  [unwired: 1 in, 1 out]
              n365 = To Unsigned Long Integer(number=w489) -> (unsigned 32bit integer=w488:u32)
              n366 = property class="Arr"(reference=w491, "Index Values"=u32[] [0, 0]) -> ()  [unwired: 1 in, 2 out]
              n367 = property class="Arr"(reference=w491, "Number of Rows"=w488) -> ()  [unwired: 1 in, 2 out]
            }
            n368 = To Double Precision Float(number=w479) -> (double precision float=w478:dbl)
            n369 = property on="Scrollbar" class="Scroll (strict)"("DocMax"=w478) -> ()  [unwired: 2 in, 2 out]
          }
        }
      }
      event "Clear layer": Value Change {
        w495 = FALSE
        # "Resets the Layer Cluster."
        n370 = event-data() -> ()  [unwired: 1 in, 6 out]
        n371 = local write "Repeats"(1) -> ()
        n372 = property on="Scrollbar" class="Scroll (strict)"("DocMax"=1.0) -> ()  [unwired: 2 in, 2 out]
        n373 = property on="add_modify" class="Bool"("Disabled"=2) -> ()  [unwired: 2 in, 2 out]
        n374 = local write "Layer Cluster"(cluster{bool[], u16[][], bool[], sgl[]} {[FALSE], [[0, 0, 0, 0]], [FALSE], [0.0]}) -> ()
        n375 = property on="Layer Cluster" class="Clust (strict)"() -> ("Controls[]"=w499:refnum<vi>[])  [unwired: 2 in, 2 out]
        n376 = for {
          tunnel: w499 -> [w502] mode=indexing
          w503 = refnum<vi> refnum  # Array
          n377 = To More Specific Class(target class=w503, reference=w502) -> (specific class reference=w501:refnum<vi>)  [unwired: 1 in, 1 out]
          n378 = property class="Arr"(reference=w501, "Number of Rows"=u32 1) -> ()  [unwired: 1 in, 2 out]
        }
      }
      event "Clear all": Value Change {
        w504 = 2
        w509 = 1
        w508 = cluster{bool[], u16[][], bool[], sgl[]} {[FALSE], [[0, 0, 0, 0]], [FALSE], [0.0]}
        w512 = FALSE
        # "Resets the GUI and the Output Array."
        n379 = event-data() -> ()  [unwired: 1 in, 6 out]
        n380 = Bundle(w508, w509) -> (w510:T12)  [unwired: 1 in]
        n381 = local write "Layer Cluster"(w508) -> ()
        n382 = local write "Temp"(w510) -> ()
        n383 = local write "Repeats"(w509) -> ()
        n384 = local write "Output Array"(cluster{u16[][], bool[], sgl[], i32}[] []) -> ()
        n385 = property on="Sequence" class="MCListbox (strict)"("ItemNames"=string[][] []) -> ()  [unwired: 2 in, 2 out]
        n386 = property on="Scrollbar" class="Scroll (strict)"("DocMax"=1.0) -> ()  [unwired: 2 in, 2 out]
        n387 = property on="Layer Cluster" class="Clust (strict)"() -> ("Controls[]"=w506:refnum<vi>[])  [unwired: 2 in, 2 out]
        n388 = for {
          tunnel: w506 -> [w516] mode=indexing
          w517 = refnum<vi> refnum  # Array
          n389 = To More Specific Class(target class=w517, reference=w516) -> (specific class reference=w514:refnum<vi>)  [unwired: 1 in, 1 out]
          n390 = property class="Arr"(reference=w514, "Number of Rows"=u32 1) -> ()  [unwired: 1 in, 2 out]
          n391 = property class="Arr"(reference=w514, "Index Values"=u32[] [0, 0]) -> ()  [unwired: 1 in, 2 out]
        }
        n392 = property on="up" class="Bool"("Disabled"=w504) -> ()  [unwired: 2 in, 2 out]
        n393 = property on="down" class="Bool"("Disabled"=w504) -> ()  [unwired: 2 in, 2 out]
        n394 = property on="Start" class="Bool"("Disabled"=w504) -> ()  [unwired: 2 in, 2 out]
        n395 = property on="add_modify" class="Bool"("Disabled"=w504) -> ()  [unwired: 2 in, 2 out]
        n396 = property on="delete_cancel" class="Bool"("Disabled"=w504) -> ()  [unwired: 2 in, 2 out]
      }
      event "Output Array": Value Change {
        w518 = FALSE
        # "Activates/deactivates the Start button if the Output Array is populated/empty."
        n397 = event-data() -> ()  [unwired: 1 in, 6 out]
        n398 = local read "Output Array"() -> (w524:T2)
        n399 = Array Size(array=w524) -> (size(s)=w523:i32)
        n400 = Equal To 0?(x=w523) -> (x = 0?=w519:bool)
        n401 = Boolean To (0,1)(Boolean=w519) -> (0, 1=w520:i16)
        n402 = Multiply(x=i16 2, y=w520) -> (x*y=w522:i16)
        n403 = property on="Start" class="Bool"("Disabled"=w522) -> ()  [unwired: 2 in, 2 out]
      }
    }
    n404 = local read "Output Array"() -> (w52:T2)
    "error out" <- w55
  }
  "Start/Cancel" <- w5
  "# of layers" <- w4
  "Output Array" <- w1
